vi "4-channel oscilloscope v1.2.vi"() -> ()   [LabVIEW 2014]
doc: "This example shows how to configure multiple channels and acquire waveforms from multiple channels."
uses:
  <vilib>/Analysis/baseanly.llb/Mean (DBL).vi
  <instrlib>/Tektronix TDS 200 1000 2000 Series/Tektronix TDS 200 1000 2000 Series.lvlib
  <vilib>/Analysis/NI_AALBase.lvlib
panel:
  out "Ch4":dbl
  out "Ch3":dbl
  out "Ch2":dbl
  out "Ch1":dbl
  out "Ch4":waveform(dbl)[](graph)
  out "Ch3":waveform(dbl)[](graph)
  out "Ch2":waveform(dbl)[](graph)
  in  "Channel 4 (3: Channel 4)":u16(ring) items=["Channel 1", "Channel 2", "Channel 3", "Channel 4", "Math", "Reference A", "Reference B", "Reference C", "Reference D"]
  in  "Probe Attenuation 4 (0.1)":dbl=10.0
  in  "Vertical Coupling 4 (1: DC)":u16(ring)=1 items=["AC", "DC", "Ground"]
  in  "Channel 3 (2: Channel 3)":u16(ring) items=["Channel 1", "Channel 2", "Channel 3", "Channel 4", "Math", "Reference A", "Reference B", "Reference C", "Reference D"]
  in  "Probe Attenuation 3 (0.1)":dbl=10.0
  in  "Vertical Coupling 3 (1: DC)":u16(ring)=1 items=["AC", "DC", "Ground"]
  in  "Channel 2 (1: Channel 2)":u16(ring)=1 items=["Channel 1", "Channel 2", "Channel 3", "Channel 4", "Math", "Reference A", "Reference B", "Reference C", "Reference D"]
  in  "Channel 1 (0: Channel 1)":u16(ring) items=["Channel 1", "Channel 2", "Channel 3", "Channel 4", "Math", "Reference A", "Reference B", "Reference C", "Reference D"]
  in  "Serial Configuration":T1={"Baud Rate"=9600, "Parity"=0, "Stop Bits"=10, "Flow Control"=2} {"Flow Control" items=["None", "XON/XOFF", "RTS/CTS", "XON/XOFF & RTS/CTS", "DTR/DSR", "XON/XOFF & DTR/DSR"]; "Stop Bits" items=["1.0"=10, "1.5"=15, "2.0"=20]; "Parity" items=["None", "Odd", "Even", "Mark", "Space"]; "Baud Rate" items=["300"=300, "600"=600, "1200"=1200, "2400"=2400, "4800"=4800, "9600"=9600, "19200"=19200]}
  in  "Probe Attenuation 2 (0.1)":dbl=1.0
  in  "Vertical Coupling 2 (1: DC)":u16(ring)=1 items=["AC", "DC", "Ground"]
  in  "Probe Attenuation 1 (0.1)":dbl=10.0
  in  "Vertical Coupling 1 (1: DC)":u16(ring)=1 items=["AC", "DC", "Ground"]
  in  "Timeout (10000 ms)":u32=10000
  out "Ch1":waveform(dbl)[](graph)
  in  "VISA resource name":refnum<visa-resource-name>
  # "2015 NanoBEEs"
  # "Channel 3"
  # "Channel 1"
  # "Channel 2"
  # "Channel 4"
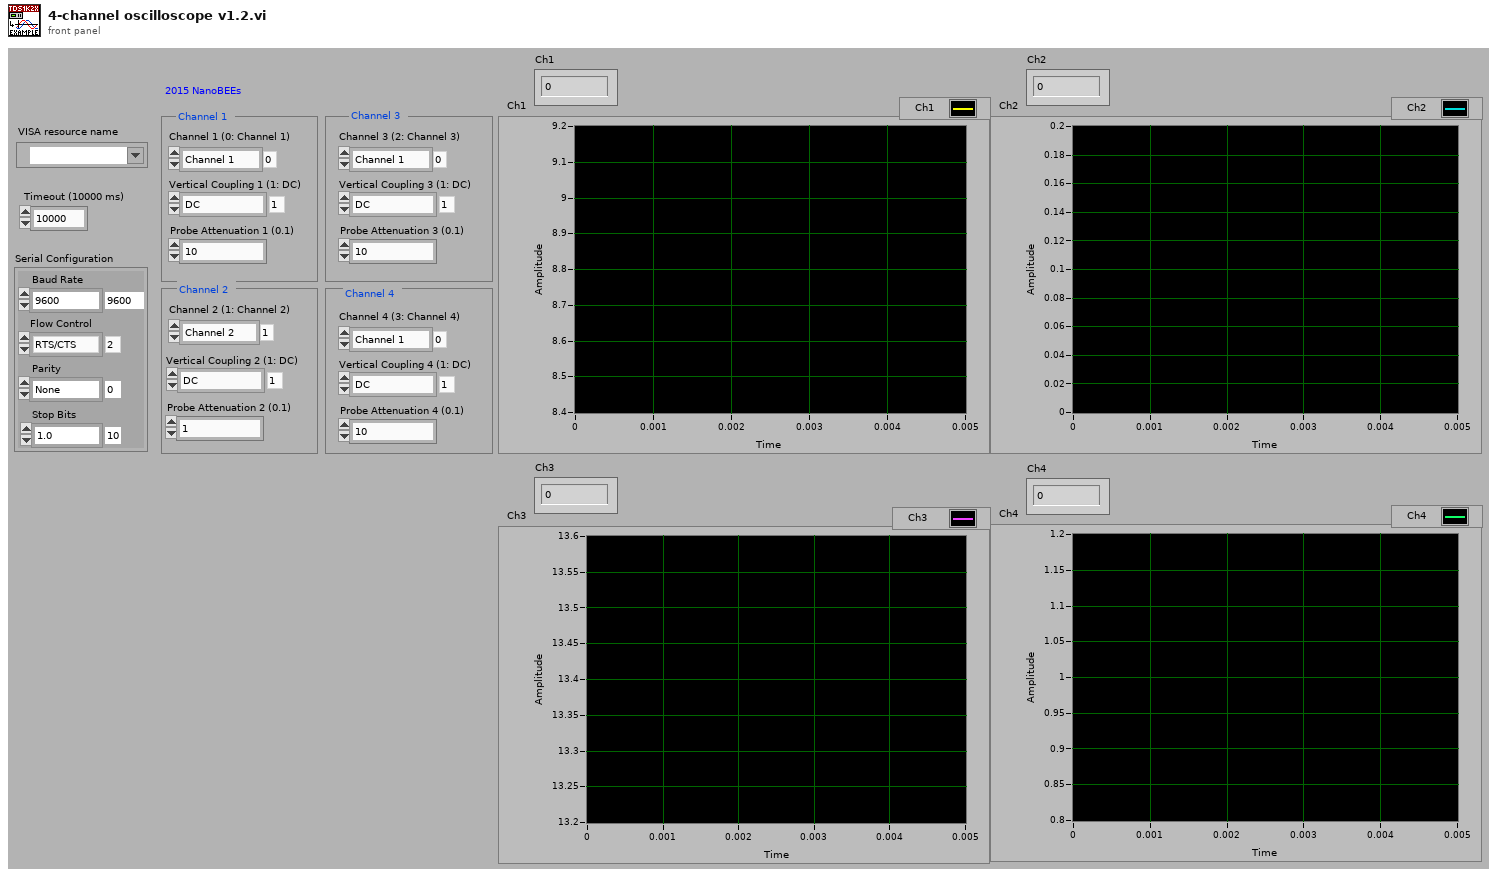
[diagram p1: front panel]
types:
  T1 = cluster{"Baud Rate":u32, "Parity":u16, "Stop Bits":u16, "Flow Control":u16}
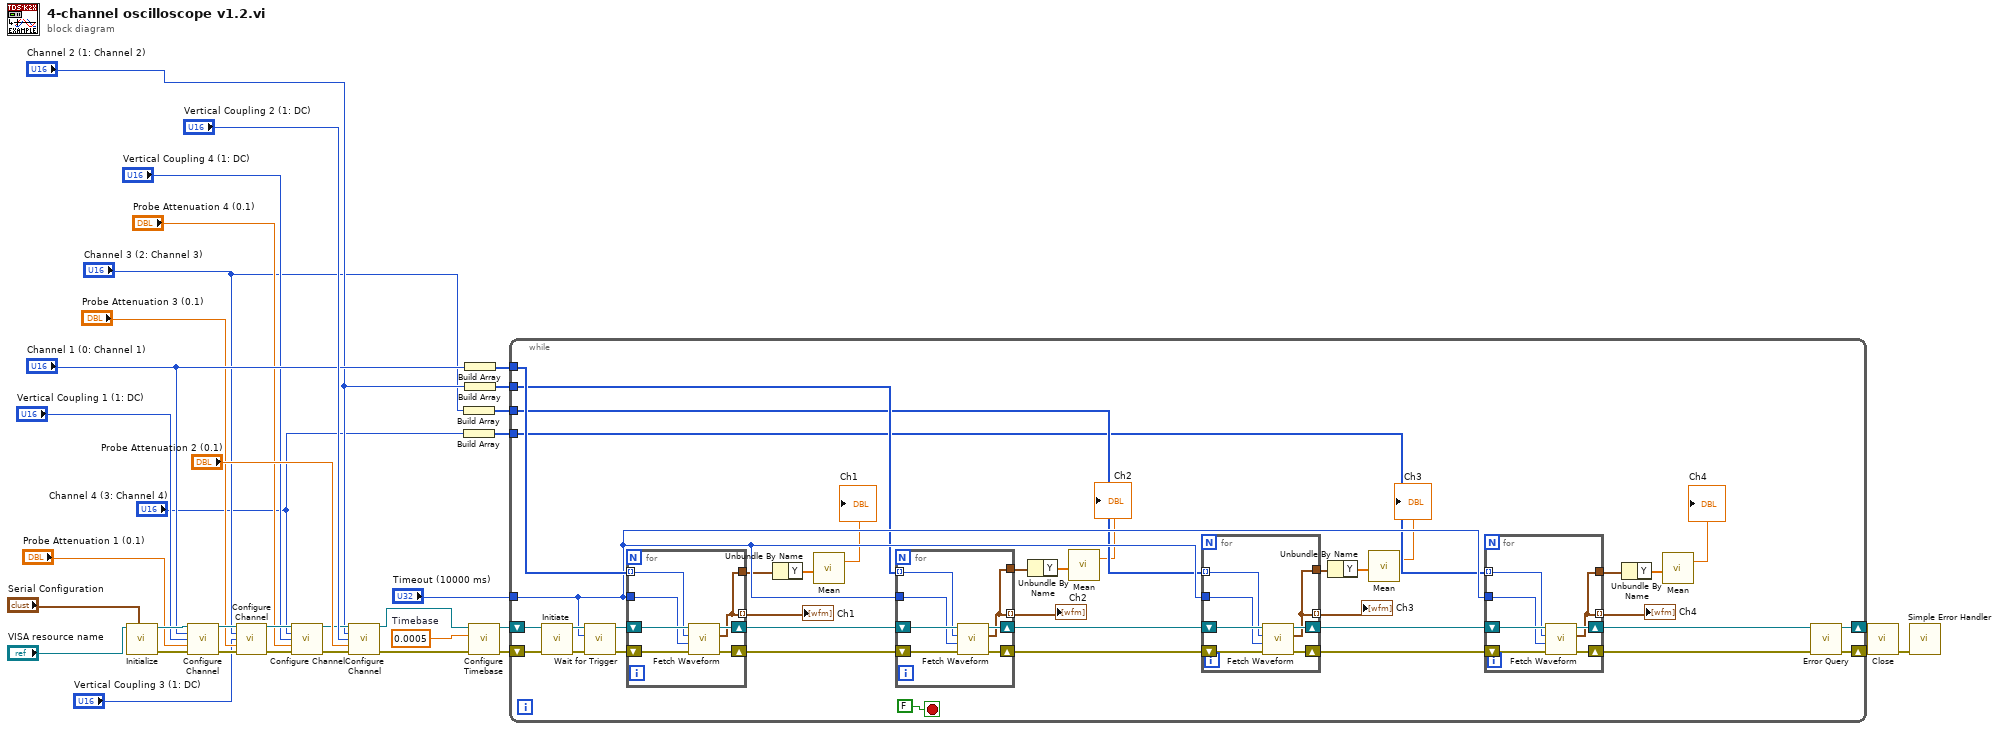
[diagram p0: block diagram]
diagram:
  w21 = 0.0005  # Timebase
  n1 = call <instrlib>:"Initialize.vi"("Serial Configuration"="Serial Configuration", "VISA resource name"="VISA resource name") -> ("error out"=w30:errorcluster, "VISA resource name out"=w31:refnum<visa-resource-name>)  [unwired: 3 in, 5 out]
  n2 = call <instrlib>:"Configure Channel.vi"("VISA resource name"=w31, "Channel (0: Channel 1)"="Channel 1 (0: Channel 1)", "Vertical Coupling (1: DC)"="Vertical Coupling 1 (1: DC)", "Probe Attenuation (10: 10X)"="Probe Attenuation 1 (0.1)", "error in (no error)"=w30) -> ("VISA resource name out"=w16:refnum<visa-resource-name>, "error out"=w13:errorcluster)  [unwired: 4 in, 5 out]
  n3 = call <instrlib>:"Configure Channel.vi"("VISA resource name"=w16, "Channel (0: Channel 1)"="Channel 3 (2: Channel 3)", "Vertical Coupling (1: DC)"="Vertical Coupling 3 (1: DC)", "Probe Attenuation (10: 10X)"="Probe Attenuation 3 (0.1)", "error in (no error)"=w13) -> ("VISA resource name out"=w15:refnum<visa-resource-name>, "error out"=w12:errorcluster)  [unwired: 4 in, 5 out]
  n4 = call <instrlib>:"Configure Channel.vi"("VISA resource name"=w15, "Channel (0: Channel 1)"="Channel 4 (3: Channel 4)", "Vertical Coupling (1: DC)"="Vertical Coupling 4 (1: DC)", "Probe Attenuation (10: 10X)"="Probe Attenuation 4 (0.1)", "error in (no error)"=w12) -> ("VISA resource name out"=w14:refnum<visa-resource-name>, "error out"=w11:errorcluster)  [unwired: 4 in, 5 out]
  n5 = call <instrlib>:"Configure Channel.vi"("VISA resource name"=w14, "Channel (0: Channel 1)"="Channel 2 (1: Channel 2)", "Vertical Coupling (1: DC)"="Vertical Coupling 2 (1: DC)", "Probe Attenuation (10: 10X)"="Probe Attenuation 2 (0.1)", "error in (no error)"=w11) -> ("VISA resource name out"=w29:refnum<visa-resource-name>, "error out"=w28:errorcluster)  [unwired: 4 in, 5 out]
  n6 = Build Array("Channel 3 (2: Channel 3)") -> (w2:u16[])
  n7 = Build Array("Channel 4 (3: Channel 4)") -> (w1:u16[])
  n8 = Build Array("Channel 1 (0: Channel 1)") -> (w20:u16[])
  n9 = Build Array("Channel 2 (1: Channel 2)") -> (w5:u16[])
  n10 = call <instrlib>:"Configure Timebase.vi"("error in (no error)"=w28, "Timebase (0.0005 s)"=w21, "VISA resource name"=w29) -> ("error out"=w26:errorcluster, "VISA resource name out"=w27:refnum<visa-resource-name>)  [unwired: 1 in, 6 out]
  n11 = while {
    tunnel: w20 -> [w52]
    tunnel: "Timeout (10000 ms)" -> [w51]
    shift-right: [w66] -> w33
    shift-left: w27 -> [w68]
    shift-right: [w65] -> w32
    shift-left: w26 -> [w67]
    tunnel: w5 -> [w50]
    tunnel: w2 -> [w49]
    tunnel: w1 -> [w48]
    stop <- FALSE stop-if-true
    n12 = call <instrlib>:"Initiate.vi"("error in (no error)"=w67, "VISA resource name"=w68) -> ("error out"=w69:errorcluster, "VISA resource name out"=w72:refnum<visa-resource-name>)  [unwired: 8 out]
    n13 = call <instrlib>:"Wait for Trigger.vi"("error in (no error)"=w69, "Timeout (10000 ms)"=w51, "VISA resource name"=w72) -> ("error out"=w70:errorcluster, "VISA resource name out"=w71:refnum<visa-resource-name>)  [unwired: 7 out]
    n14 = for {
      shift-right: [w100] -> w62
      shift-left: w70 -> [w98]
      tunnel: w52 -> [w96] mode=indexing
      tunnel: [w95] -> w64 mode=indexing
      tunnel: w51 -> [w97]
      shift-right: [w101] -> w63
      shift-left: w71 -> [w99]
      tunnel: [w95] -> w47
      n15 = call <instrlib>:"Fetch Waveform.vi"("error in (no error)"=w98, "Timeout (10000 ms)"=w97, "Source (0: Channel 1)"=w96, "VISA resource name"=w99) -> ("error out"=w100:errorcluster, "Waveform Data"=w95:waveform(dbl), "VISA resource name out"=w101:refnum<visa-resource-name>)  [unwired: 2 in, 3 out]
    }
    "Ch1" <- w64
    n16 = Unbundle By Name(w47) -> ("Y"=w46:dbl[])
    n17 = call-poly <vilib>:"Mean.vi"("X"=w46) -> ("mean"=→"Ch1":dbl)  [unwired: 1 out]
    n18 = for {
      shift-right: [w93] -> w53
      shift-left: w62 -> [w91]
      tunnel: w50 -> [w89] mode=indexing
      tunnel: [w88] -> w61 mode=indexing
      tunnel: w51 -> [w90]
      shift-right: [w94] -> w54
      shift-left: w63 -> [w92]
      tunnel: [w88] -> w39
      n19 = call <instrlib>:"Fetch Waveform.vi"("error in (no error)"=w91, "Timeout (10000 ms)"=w90, "Source (0: Channel 1)"=w89, "VISA resource name"=w92) -> ("error out"=w93:errorcluster, "Waveform Data"=w88:waveform(dbl), "VISA resource name out"=w94:refnum<visa-resource-name>)  [unwired: 2 in, 3 out]
    }
    "Ch2" <- w61
    n20 = Unbundle By Name(w39) -> ("Y"=w38:dbl[])
    n21 = call-poly <vilib>:"Mean.vi"("X"=w38) -> ("mean"=→"Ch2":dbl)  [unwired: 1 out]
    n22 = for {
      shift-right: [w86] -> w57
      shift-left: w53 -> [w84]
      tunnel: w49 -> [w82] mode=indexing
      tunnel: [w81] -> w60 mode=indexing
      tunnel: w51 -> [w83]
      shift-right: [w87] -> w58
      shift-left: w54 -> [w85]
      tunnel: [w81] -> w40
      n23 = call <instrlib>:"Fetch Waveform.vi"("error in (no error)"=w84, "Timeout (10000 ms)"=w83, "Source (0: Channel 1)"=w82, "VISA resource name"=w85) -> ("error out"=w86:errorcluster, "Waveform Data"=w81:waveform(dbl), "VISA resource name out"=w87:refnum<visa-resource-name>)  [unwired: 2 in, 3 out]
    }
    "Ch3" <- w60
    n24 = Unbundle By Name(w40) -> ("Y"=w37:dbl[])
    n25 = call-poly <vilib>:"Mean.vi"("X"=w37) -> ("mean"=→"Ch3":dbl)  [unwired: 1 out]
    n26 = for {
      shift-right: [w79] -> w55
      shift-left: w57 -> [w77]
      tunnel: w48 -> [w75] mode=indexing
      tunnel: [w74] -> w59 mode=indexing
      tunnel: w51 -> [w76]
      shift-right: [w80] -> w56
      shift-left: w58 -> [w78]
      tunnel: [w74] -> w41
      n27 = call <instrlib>:"Fetch Waveform.vi"("error in (no error)"=w77, "Timeout (10000 ms)"=w76, "Source (0: Channel 1)"=w75, "VISA resource name"=w78) -> ("error out"=w79:errorcluster, "Waveform Data"=w74:waveform(dbl), "VISA resource name out"=w80:refnum<visa-resource-name>)  [unwired: 2 in, 3 out]
    }
    "Ch4" <- w59
    n28 = Unbundle By Name(w41) -> ("Y"=w36:dbl[])
    n29 = call-poly <vilib>:"Mean.vi"("X"=w36) -> ("mean"=→"Ch4":dbl)  [unwired: 1 out]
    n30 = call <instrlib>:"Error Query.vi"("error in (no error)"=w55, "VISA resource name"=w56) -> ("error out"=w65:errorcluster, "VISA resource name out"=w66:refnum<visa-resource-name>)  [unwired: 8 out]
  }
  n31 = call <instrlib>:"Close.vi"("error in (no error)"=w32, "VISA resource name"=w33) -> ("error out"=w34:errorcluster)  [unwired: 9 out]
  n32 = call <vilib>:"Simple Error Handler.vi"("error in (no error)"=w34) -> ()  [unwired: 1 in, 8 out]
